vi "tb_09-Fr.vi"(0 "Etude":T2, 1 "Aff ?":bool, 5 "VS":T4, 7 "ent-2D":string[][](array[string]), 9 "do-2D":string[][](array[string]), 11 "tb in ?":bool[](array[boolean])) -> (4 "Etude":T2, 6 "VS":T4, 8 "ent-2D":T1[][](array[typedef]), 10 "do-2D":string[][](array[string]), 12 "F rep":string[](array[string]), 13 "F rep-ent":T1, 14 "F rep-lib":T1, 15 "tb in ?":bool[](array[boolean]))   [LabVIEW 2010, in "lv_04.lvlib"]
uses:
  lv_04/lv_04.lvlib
  lv_04/commandes/cX.ctl
  lv_04/commandes/cSTA_varid.ctl
  lv_04/commandes/c_TDMS_ch_variable.ctl
  lv_04/commandes/c_TDMS_ch_donnees.ctl
  lv_04/commandes/c0-var-n.ctl
  lv_04/commandes/cSTA_num_do_cr.ctl
  lv_04/commandes/c02-do-num.ctl
  lv_04/commandes/c04-stat-num.ctl
  lv_04/commandes/cSTA_txt_do_cr.ctl
  lv_04/commandes/c02-do-txt.ctl
  lv_04/commandes/c04-stat-txt.ctl
  lv_04/commandes/cSTA_dist.ctl
  lv_04/commandes/c03-dist-S.ctl
  lv_04/commandes/c0-dist-xy.ctl
  lv_04/commandes/c03-dist-T.ctl
  lv_04/commandes/c03-dist-SPC.ctl
  lv_04/commandes/c_etude.ctl
  lv_02/p_5E_ch_loi.ctl
  lv_01/type format.ctl
  lv_01/lv_01.lvlib
  lv_02/lv_02.lvlib
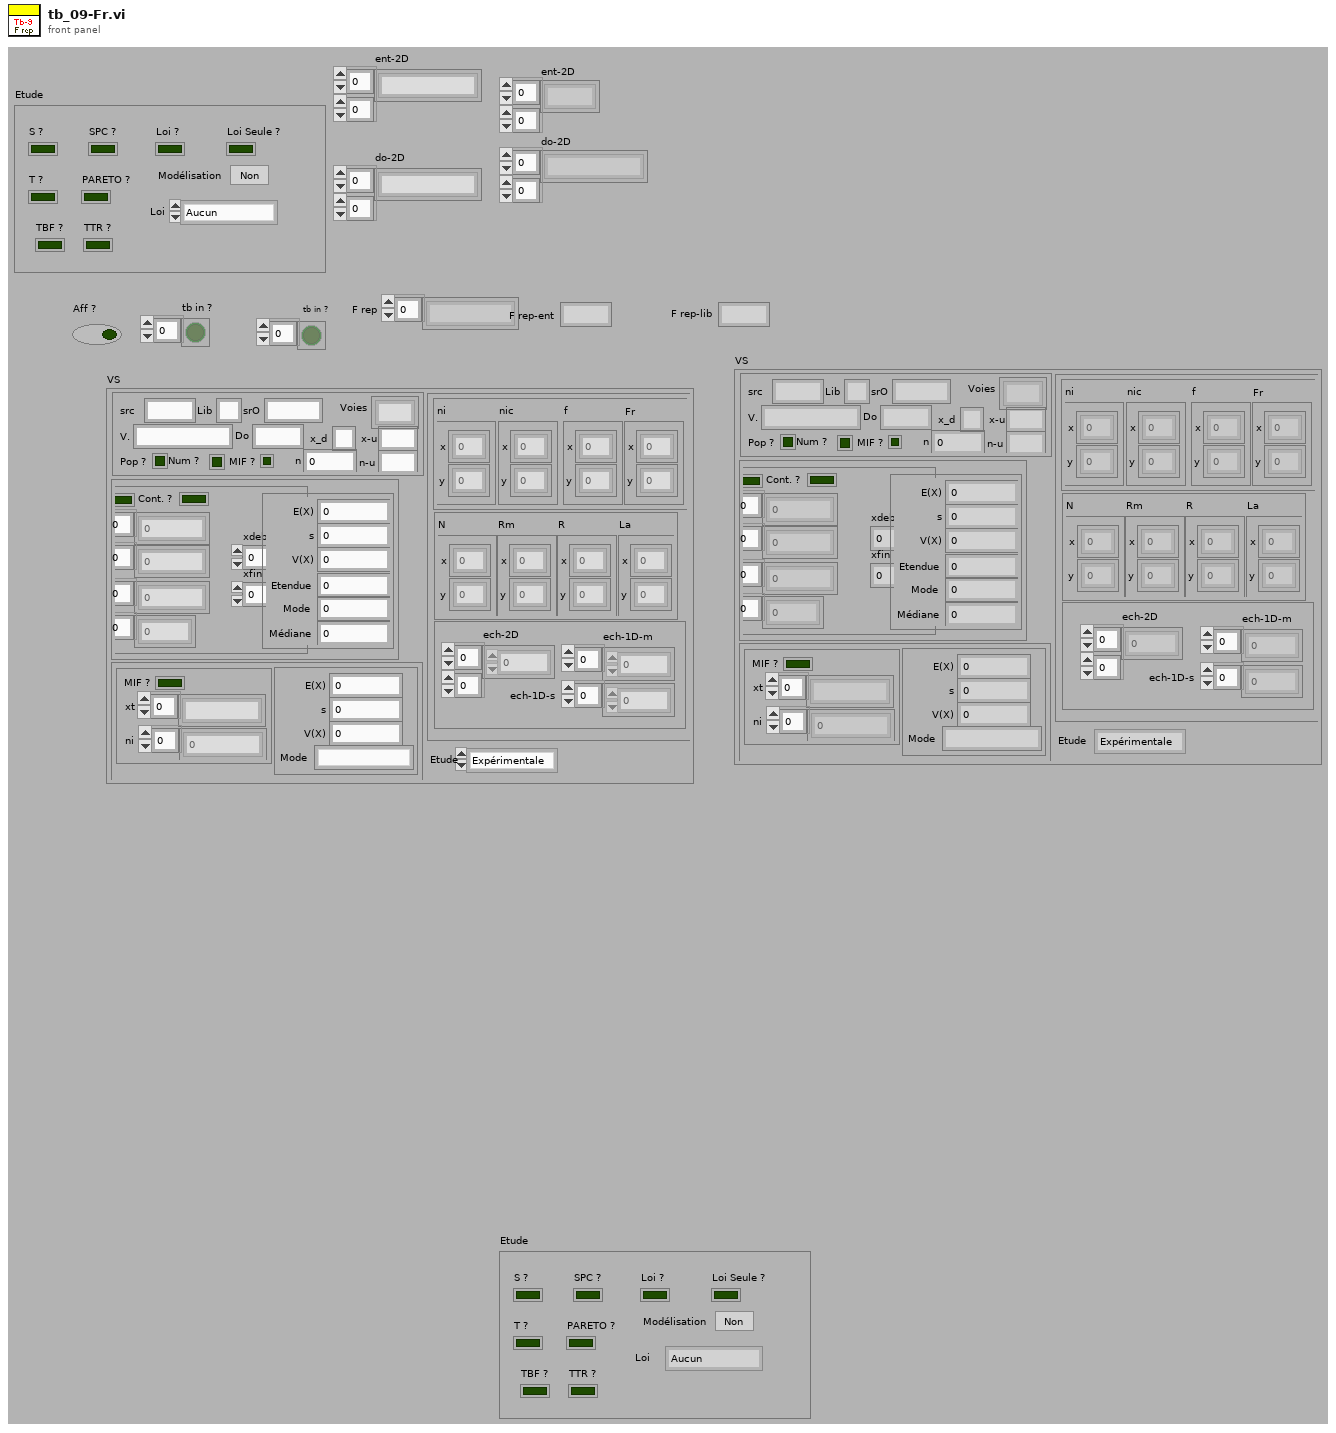
[diagram p1: front panel]
types:
  T1 = typedef "lv_04.lvlib/c_TDMS_ch_donnees.ctl" = string
  T2 = typedef "lv_04.lvlib/c_etude.ctl" = cluster{"T ?":bool, "S ?":bool, "SPC ?":bool, "PARETO ?":bool, "TBF ?":bool, "TTR ?":bool, "Loi ?":bool, "Loi Seule ?":bool, "Modélisation":bool, "Loi":T3}
  T3 = typedef "lv_02.lvlib/p_5E_ch_loi.ctl" = enum16{"Aucun", "Normale", "Aucun2", "Aucun3", "Binômial", "Poisson", "Exponentiel", "Weibull", "Rang médian"}
  T4 = typedef "lv_04.lvlib/cX.ctl" = cluster{"src":T5, "num":T8, "txt":T11, "dist":T14, "Etude":enum16{"Expérimentale", "Modèle"}}
  T5 = typedef "lv_04.lvlib/cSTA_varid.ctl" = cluster{"src":string, "Lib":string, "srO":string, "V.":T6, "Voies":string[], "Do":T1, "n":T7, "Num ?":bool, "Pop ?":bool, "x_d":string, "x-u":string, "n-u":string, "MIF ?":bool}
  T6 = typedef "lv_04.lvlib/c_TDMS_ch_variable.ctl" = string
  T7 = typedef "lv_04.lvlib/c0-var-n.ctl" = i32
  T8 = typedef "lv_04.lvlib/cSTA_num_do_cr.ctl" = cluster{"do":T9, "sta":T10}
  T9 = typedef "lv_04.lvlib/c02-do-num.ctl" = cluster{"MIF ?":bool, "Cont. ?":bool, "xi":dbl[], "xic":dbl[], "ni":u32[], "dx":dbl[], "xdeb":dbl, "xfin":dbl}
  T10 = typedef "lv_04.lvlib/c04-stat-num.ctl" = cluster{"E(X)":dbl, "s":dbl, "V(X) ":dbl, "Etendue":dbl, "Mode":dbl, "Médiane":dbl}
  T11 = typedef "lv_04.lvlib/cSTA_txt_do_cr.ctl" = cluster{"do":T12, "sta":T13}
  T12 = typedef "lv_04.lvlib/c02-do-txt.ctl" = cluster{"xt":string[], "ni":dbl[], "MIF ?":bool}
  T13 = typedef "lv_04.lvlib/c04-stat-txt.ctl" = cluster{"E(X)":dbl, "s":dbl, "V(X) ":dbl, "Mode":string}
  T14 = typedef "lv_04.lvlib/cSTA_dist.ctl" = cluster{"S":T15, "T":T17, "spc":T18}
  T15 = typedef "lv_04.lvlib/c03-dist-S.ctl" = cluster{"nic":T16, "f":T16, "Fr":T16, "ni":T16}
  T16 = typedef "lv_04.lvlib/c0-dist-xy.ctl" = cluster{"x":dbl[], "y":dbl[]}
  T17 = typedef "lv_04.lvlib/c03-dist-T.ctl" = cluster{"N":T16, "Rm":T16, "R":T16, "La":T16}
  T18 = typedef "lv_04.lvlib/c03-dist-SPC.ctl" = cluster{"ech-2D":dbl[][], "ech-1D-m":dbl[], "ech-1D-s":dbl[]}
  T19 = typedef "lv_01.lvlib/type format.ctl" = enum16{"X (dbl)", "P (Proba)", "N (entier)", "S (Scient.)"}
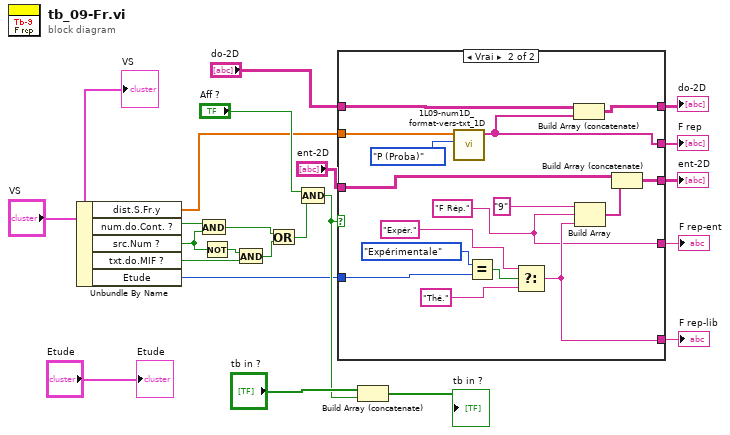
[diagram p0: block diagram]
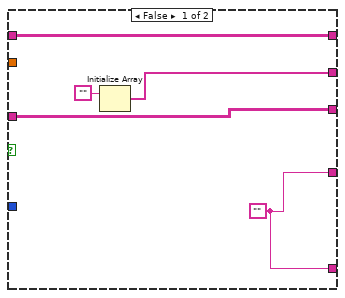
[diagram p2: hidden frame]
diagram:
  n1 = Unbundle By Name("VS") -> ("dist.S.Fr.y"=w10:dbl[], "num.do.Cont. ?"=w7:bool, "src.Num ?"=w6:bool, "txt.do.MIF ?"=w4:bool, "Etude"=w8:enum16{"Expérimentale", "Modèle"})
  n2 = And(x=w7, y=w6) -> (x .and. y?=w2:bool)
  n3 = Not(x=w6) -> (.not. x?=w5:bool)
  n4 = And(x=w5, y=w4) -> (x .and. y?=w3:bool)
  n5 = Or(x=w2, y=w3) -> (x .or. y?=w1:bool)
  n6 = Compound Arithmetic op=AND("Aff ?", w1) -> (w12:bool)
  n7 = case shown="Vrai" w12 {
    tunnel: w10 -> [_ w37]
    tunnel: [w27 w35] -> w21
    tunnel: "do-2D" -> [w25 w43]
    tunnel: [w25 w42] -> w19
    tunnel: "ent-2D" -> [w24 w41]
    tunnel: [w24 w39] -> w17
    tunnel: [w23 w33] -> w16
    tunnel: [w23 w34] -> w15
    tunnel: w8 -> [_ w30]
    frame False {
      w23 = ""
      n8 = Initialize Array("") -> (w27:string[])  [unwired: 1 in]
    }
    frame True {
      w33 = "F Rép."
      n9 = call "1L09-num1D_format-vers-txt_1D.vi"("type"=type_format."P (Proba)", "1D( num)"=w37) -> ("1D (ch)"=w35:string[])  [unwired: 7 in]
      n10 = Equal?(x=enum16{"Expérimentale", "Modèle"}."Expérimentale" ("Etude"), y=w30) -> (x = y?=w32:bool)
      n11 = Select(t="Expér.", s=w32, f="Thé.") -> (s? t:f=w34:string)
      n12 = Build Array (concatenate)(w43, w35) -> (w42:string[][])
      n13 = Build Array("9", w33, w34) -> (w40:string[])
      n14 = Build Array (concatenate)(w41, w40) -> (w39:string[][])
    }
  }
  "F rep" <- w21
  "F rep-ent" <- w16
  "F rep-lib" <- w15
  "ent-2D" <- w17
  "do-2D" <- w19
  n15 = Build Array (concatenate)("tb in ?", w12) -> (→"tb in ?":bool[])
  "VS" <- "VS"
  "Etude" <- "Etude"
